vi "System@RecordSave__Parameter.vi"(1 "ParamterIn":string) -> (0 "ParamterOut":string)   [LabVIEW 2019]
panel:
  in  "Message":string(combo)
  in  "Record":string(combo)
  in  "Confirm":bool
  # "System@RecordSave $Record,$RecordFile"
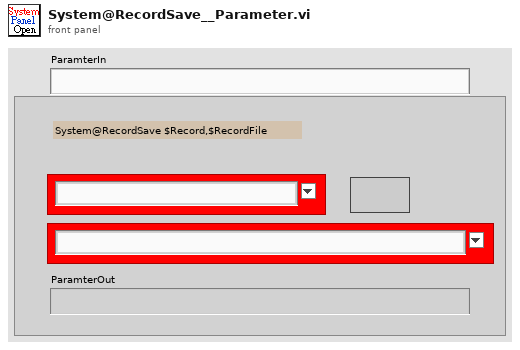
[diagram p1: front panel]
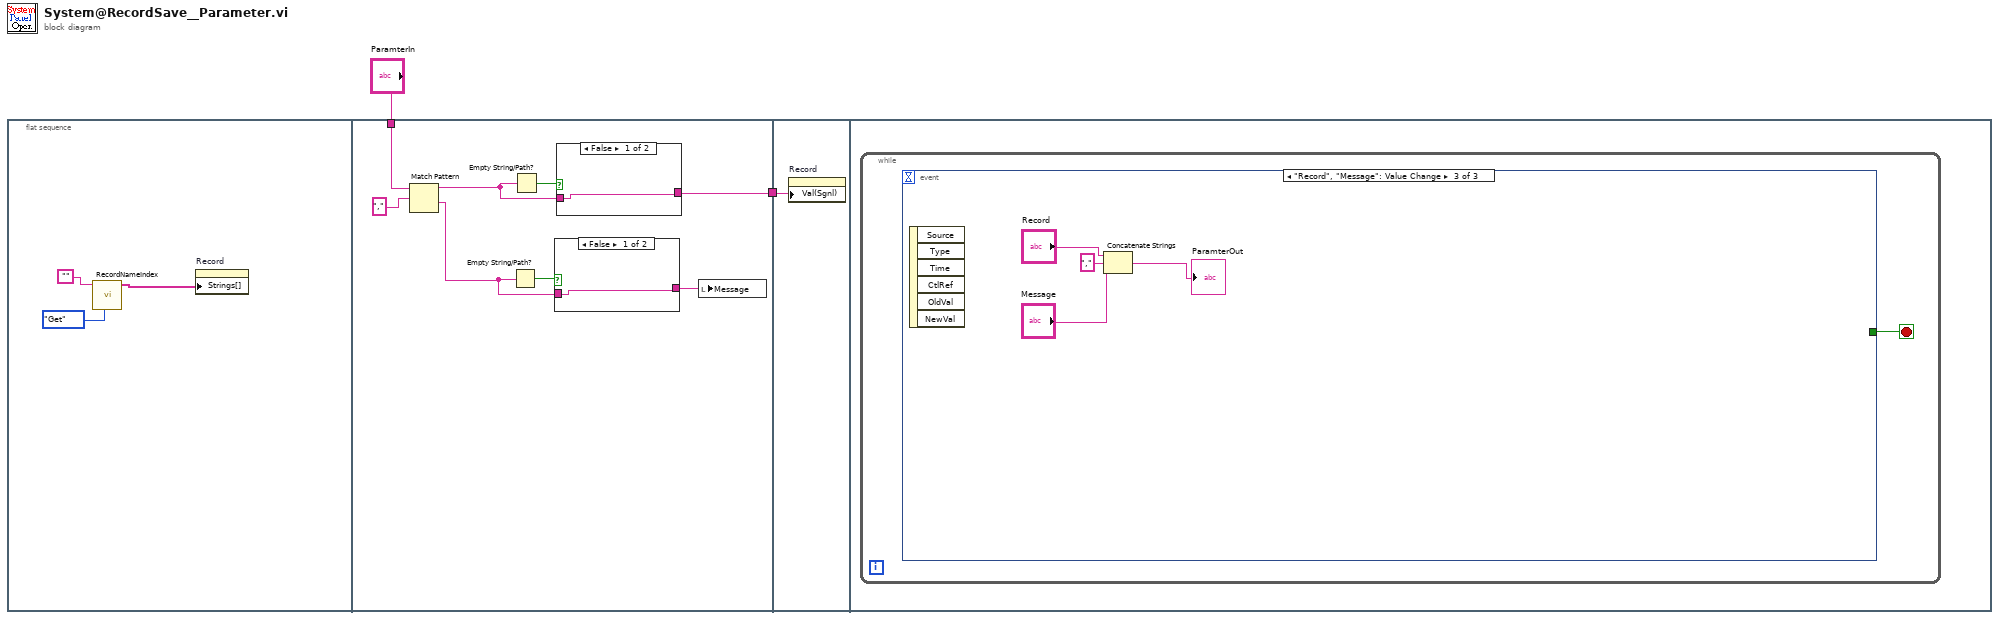
[diagram p0: block diagram]
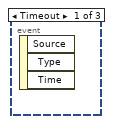
[diagram p4: hidden frame]
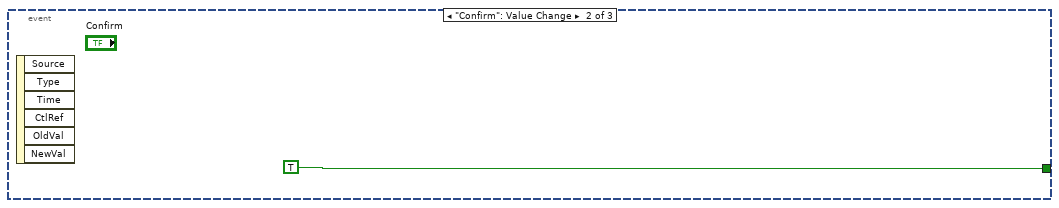
[diagram p5: hidden frame]
diagram:
  n1 = flat-sequence {
    tunnel: "ParamterIn" -> [w12]
    tunnel: [w7] -> w1
    tunnel: w1 -> [w18]
    frame #0 {
      n2 = call "RecordNameIndex.vi"("OP"=enum16{"Init", "Insert", "Get", "Write"}."Get", "ItemCatalog"="") -> ("NamelList"=w4:string[])  [unwired: 6 in, 3 out]
      n3 = property on="Record" class="CmbBox"("Strings[]"=w4) -> ()  [unwired: 2 in, 2 out]
    }
    frame #1 {
      n4 = Match Pattern(string=w12, regular expression=",") -> (before substring=w10:string, after substring=w8:string)  [unwired: 1 in, 2 out]
      n5 = Empty String/Path?(string/path=w8) -> (empty?=w9:bool)
      n6 = Empty String/Path?(string/path=w10) -> (empty?=w13:bool)
      n7 = case shown="False" w9 {
        tunnel: w8 -> [w14 w15]
        tunnel: [w14 w15] -> w6
        frame False {
        }
        frame True {
        }
      }
      n8 = case shown="False" w13 {
        tunnel: w10 -> [w16 w17]
        tunnel: [w16 w17] -> w7
        frame False {
        }
        frame True {
        }
      }
      n9 = local write "Message"(w6) -> ()
    }
    frame #2 {
      n10 = property on="Record" class="CmbBox"("Val(Sgnl)"=w18) -> ()  [unwired: 2 in, 2 out]
    }
    frame #3 {
      n11 = while {
        stop <- w19 stop-if-true
        n12 = event shown="[2] \"Record\", \"Message\": Value Change" {
          selector: _ -> [_ _ _]
          dyn-events: _ -> [_ _ _]
          timeout: _ -> [_ _ _]
          tunnel: [_ TRUE _] -> w19
          event Timeout {
            n13 = event-data() -> ()  [unwired: 1 in, 3 out]
          }
          event "Confirm": Value Change {
            n14 = event-data() -> ()  [unwired: 1 in, 6 out]
          }
          event "Record", "Message": Value Change {
            n15 = event-data() -> ()  [unwired: 1 in, 6 out]
            n16 = Concatenate Strings("Record", "," ("string"), "Message") -> (→"ParamterOut":string)
          }
        }
      }
    }
  }
